vi "Setup file input channels.vi"(8 "error in":errorcluster, 9 "Sampling data":T1={"Channels"=[], "Sampling freq"=0.0, "Output freq"=0.0, "Update freq"=0.0, "Steps per rev"=0, "Counts per rev"=0, "Amplifier"="", "Motor driver"="", "Step bit"=0, "Max speed"=0.0, "Max accel"=0.0, "Pos gain"=0.0, "Vel gain"=0.0, "counter"="Dev1/ctr0"} {"Channels"."Hi cutoff" items=["500"=500.0, "1k"=1000.0, "5k"=5000.0, "10k"=10000.0, "20k"=20000.0]; "Channels"."Lo cutoff" items=["0.1"=0.1, "1"=1.0, "10"=10.0, "100"=100.0, "300"=300.0]; "Channels"."Gain" items=["x100"=100, "x1000"=1000, "x10000"=10000]}, 11 "file ref in":T3 format="%.0x") -> (0 "error out":errorcluster, 1 "Sampling data out":T1={"Channels"=[], "Sampling freq"=0.0, "Output freq"=0.0, "Update freq"=0.0, "Steps per rev"=0, "Counts per rev"=0, "Amplifier"="", "Motor driver"="", "Step bit"=0, "Max speed"=0.0, "Max accel"=0.0, "Pos gain"=0.0, "Vel gain"=0.0, "counter"="Dev1/ctr0"} {"Channels"."Hi cutoff" items=["500"=500.0, "1k"=1000.0, "5k"=5000.0, "10k"=10000.0, "20k"=20000.0]; "Channels"."Lo cutoff" items=["0.1"=0.1, "1"=1.0, "10"=10.0, "100"=100.0, "300"=300.0]; "Channels"."Gain" items=["x100"=100, "x1000"=1000, "x10000"=10000]}, 2 "dset ref":i32, 3 "file ref out":T3 format="%.0x", 4 "encoder dset":i32)   [LabVIEW 2013]
uses:
  <vilib>/addons/h5labview2/base/hid_t.ctl
  Sampling info.ctl
  Channel.ctl
  <vilib>/addons/h5labview2/base/lib_path.vi
  Create HDF5 chunked dataset (2D).vi
  <vilib>/addons/h5labview2/base/H5Equery.vi
  <vilib>/addons/h5labview2/attrib/H5Awrite.llb/H5Awrite.xnode
  <vilib>/addons/h5labview2/group/H5G.lvlib
  Create HDF5 chunked dataset (1D).vi
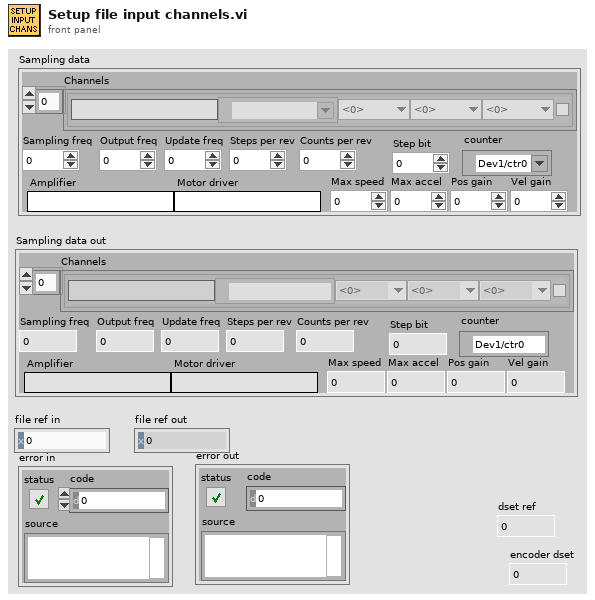
[diagram p1: front panel]
types:
  T1 = typedef "Sampling info.ctl" = cluster{"Channels":T2[], "Sampling freq":dbl, "Output freq":dbl, "Update freq":dbl, "Steps per rev":i32, "Counts per rev":i32, "Amplifier":string, "Motor driver":string, "Step bit":u8, "Max speed":dbl, "Max accel":dbl, "Pos gain":dbl, "Vel gain":dbl, "counter":tag}
  T2 = typedef "Channel.ctl" = cluster{"Name":string, "Chan":tag, "Gain":u16, "Lo cutoff":dbl, "Hi cutoff":dbl, "Notch":bool}
  T3 = typedef "hid_t.ctl" = i32
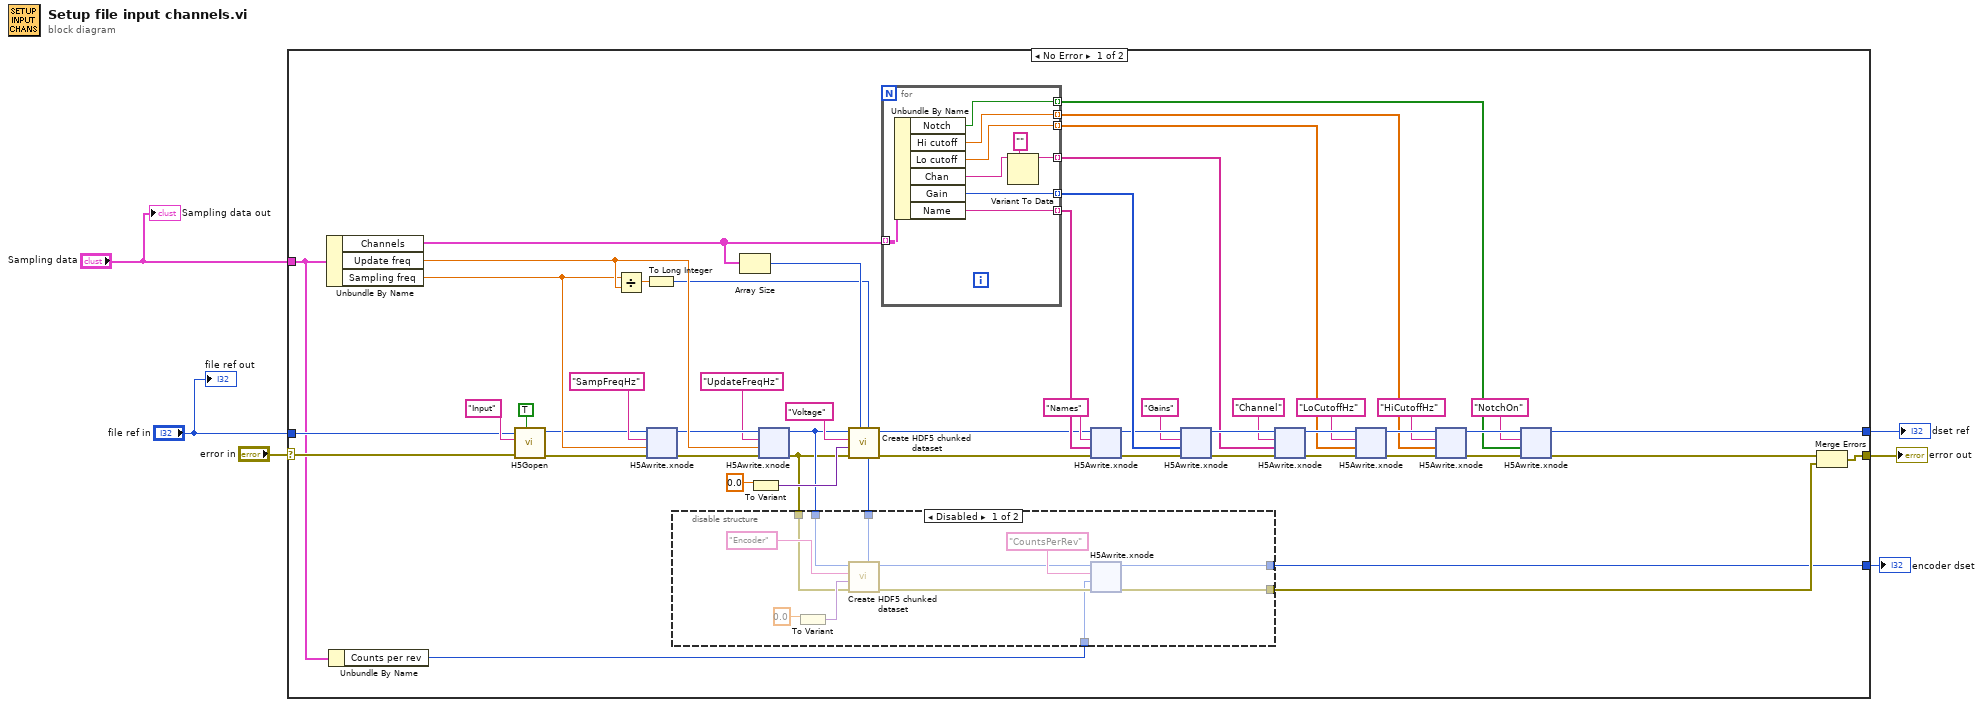
[diagram p0: block diagram]
diagram:
  n1 = case shown="No Error" "error in" {
    selector: "error in" -> [w18 w243]
    tunnel: [w58 _] -> w6
    tunnel: [w10 w243] -> w5
    tunnel: "file ref in" -> [w17 _]
    tunnel: "Sampling data" -> [w12 _]
    tunnel: [w7 _] -> w1
    frame No Error {
      n2 = Unbundle By Name(w12) -> ("Channels"=w41:T2[], "Update freq"=w37:dbl, "Sampling freq"=w36:dbl)
      n3 = Unbundle By Name(w12) -> ("Counts per rev"=w11:i32)
      n4 = call <vilib>:"H5Gopen.vi"("create? (F)"=TRUE, "error in (no error)"=w18, "name"="Input", "ref in"=w17) -> ("error out"=w23:errorcluster, "group out"=w24:T3)  [unwired: 3 in]
      n5 = Divide(x=w36, y=w37) -> (x/y=w38:dbl)
      n6 = To Long Integer(number=w38) -> (32bit integer=w13:i32)
      n7 = xnode "H5Awrite.xnode"("error in (no error)"=w23, "data"=w36, "attrib name"="SampFreqHz", "ref in"=w24) -> ("error out"=w28:errorcluster, "ref out"=w27:T3)  [unwired: 3 in, 1 out]
      n8 = Array Size(array=w41) -> (size(s)=w16:i32)
      n9 = To Variant(anything=0.0) -> (Variant=w19:variant)
      n10 = xnode "H5Awrite.xnode"("error in (no error)"=w28, "data"=w37, "attrib name"="UpdateFreqHz", "ref in"=w27) -> ("error out"=w14:errorcluster, "ref out"=w15:T3)  [unwired: 3 in, 1 out]
      n11 = disable-structure shown="Disabled" {
        disable-tunnel: w15 -> [w67 _]
        disable-tunnel: w14 -> [w66 w89]
        disable-tunnel: w13 -> [w65 _]
        disable-tunnel: w11 -> [w61 _]
        disable-tunnel: [w60 w89] -> w8
        disable-tunnel: [w59 _] -> w7
        frame Disabled {
          n12 = To Variant(anything=0.0) -> (Variant=w70:variant)
          n13 = call-poly "Create HDF5 chunked dataset.vi"("block size"=w65, "error in (no error)"=w66, "data type"=w70, "name"="Encoder", "ref in"=w67) -> ("error out"=w62:errorcluster, "dset out"=w63:i32)  [unwired: 5 in]
          n14 = xnode "H5Awrite.xnode"("error in (no error)"=w62, "data"=w61, "attrib name"="CountsPerRev", "ref in"=w63) -> ("error out"=w60:errorcluster, "ref out"=w59:T3)  [unwired: 3 in, 1 out]
        }
        frame Enabled {
        }
      }
      n15 = call-poly "Create HDF5 chunked dataset.vi"("block size"=w13, "number of channels"=w16, "error in (no error)"=w14, "data type"=w19, "name"="Voltage", "ref in"=w15) -> ("error out"=w32:errorcluster, "dset out"=w30:i32)  [unwired: 4 in]
      n16 = for {
        tunnel: w41 -> [w206] mode=indexing
        tunnel: [w205] -> w39 mode=indexing
        tunnel: [w204] -> w40 mode=indexing
        tunnel: [w201] -> w43 mode=indexing
        tunnel: [w200] -> w47 mode=indexing
        tunnel: [w199] -> w48 mode=indexing
        tunnel: [w198] -> w49 mode=indexing
        n17 = Unbundle By Name(w206) -> ("Notch"=w198:bool, "Hi cutoff"=w199:dbl, "Lo cutoff"=w200:dbl, "Chan"=w203:tag, "Gain"=w204:u16, "Name"=w205:string)
        n18 = Variant To Data(type="", Variant=w203) -> (data=w201:string)  [unwired: 1 in, 1 out]
      }
      n19 = xnode "H5Awrite.xnode"("error in (no error)"=w32, "data"=w39, "attrib name"="Names", "ref in"=w30) -> ("error out"=w35:errorcluster, "ref out"=w34:T3)  [unwired: 3 in, 1 out]
      n20 = xnode "H5Awrite.xnode"("error in (no error)"=w35, "data"=w40, "attrib name"="Gains", "ref in"=w34) -> ("error out"=w51:errorcluster, "ref out"=w50:T3)  [unwired: 3 in, 1 out]
      n21 = xnode "H5Awrite.xnode"("error in (no error)"=w51, "data"=w43, "attrib name"="Channel", "ref in"=w50) -> ("error out"=w53:errorcluster, "ref out"=w52:T3)  [unwired: 3 in, 1 out]
      n22 = xnode "H5Awrite.xnode"("error in (no error)"=w53, "data"=w47, "attrib name"="LoCutoffHz", "ref in"=w52) -> ("error out"=w55:errorcluster, "ref out"=w54:T3)  [unwired: 3 in, 1 out]
      n23 = xnode "H5Awrite.xnode"("error in (no error)"=w55, "data"=w48, "attrib name"="HiCutoffHz", "ref in"=w54) -> ("error out"=w56:errorcluster, "ref out"=w57:T3)  [unwired: 3 in, 1 out]
      n24 = xnode "H5Awrite.xnode"("error in (no error)"=w56, "data"=w49, "attrib name"="NotchOn", "ref in"=w57) -> ("error out"=w9:errorcluster, "ref out"=w58:T3)  [unwired: 3 in, 1 out]
      n25 = Merge Errors(w9, w8) -> (w10:errorcluster)
    }
    frame Error {
    }
  }
  "dset ref" <- w6
  "error out" <- w5
  "encoder dset" <- w1
  "file ref out" <- "file ref in"
  "Sampling data out" <- "Sampling data"
